vi "Digital Port Test.vi"() -> ()   [LabVIEW 2025]
doc: "Author: Scott Hannahs <sth@magnet.fsu.edu>\n\nThis software is licensed for use under the “MIT License\"\nCopyright (c) 2025 Scott Hannahs, sth@sth@magnet.sthnet.net\n\nPermission is hereby granted, free of charge, to any person obtaining a copy of this software and associated documentation files (the \"Software\"), to deal in the Software without restriction, including without limitation the rights to use, copy, modify, merge, publish, distribute, sublicense, and/or sell copies of the Software, and to permit persons to whom the Software is furnished to do so, subject to the following conditions: The above copyright notice and this permission notice shall be included in all copies or substantial portions of the Software.\n\nTHE SOFTWARE IS PROVIDED \"AS IS\", WITHOUT WARRANTY OF ANY KIND, EXPRESS OR IMPLIED, INCLUDING BUT NOT LIMITED TO THE WARRANTIES OF MERCHANTABILITY, FITNESS FOR A PARTICULAR PURPOSE AND NONINFRINGEMENT. IN NO EVENT SHALL THE AUTHORS OR COPYRIGHT HOLDERS BE LIABLE FOR ANY CLAIM, DAMAGES OR OTHER LIABILITY, WHETHER IN AN ACTION OF CONTRACT, TORT OR OTHERWISE, ARISING FROM, OUT OF OR IN CONNECTION WITH THE SOFTWARE OR THE USE OR OTHER DEALINGS IN THE SOFTWARE."
uses:
  <vilib>/Utility/error.llb/DialogType.ctl
  <vilib>/_DAQmxBase/Internals/DAQmxBase Create Channel (DO-Digital Output).vi
  <vilib>/_DAQmxBase/Internals/DAQmxBase Write (Digital U8 1Chan 1Samp).vi
panel:
  in  "stop":bool
  out "Data Read":u8 caption="Data Write" format="%02x"
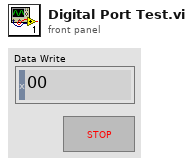
[diagram p1: front panel]
types:
  T1 = typedef "DialogType.ctl" = u16
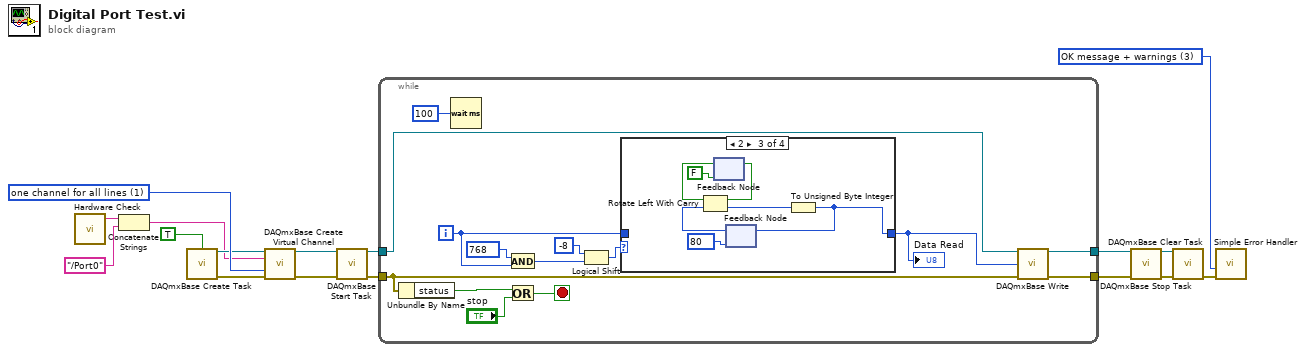
[diagram p0: block diagram]
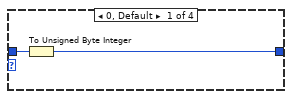
[diagram p2: hidden frame]
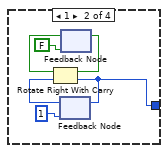
[diagram p3: hidden frame]
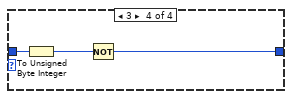
[diagram p4: hidden frame]
diagram:
  w11 = 1 items=["one channel for each line", "one channel for all lines"] ("line grouping")
  w12 = T1 3 items=["no dialog", "OK message", "continue or stop message", "OK message + warnings", "continue/stop + warnings"] ("type of dialog (OK msg:1)")
  n1 = call "Hardware Check.vi"() -> ("Data Acq Device"=w4:string)  [unwired: 1 in, 2 out]
  n2 = Concatenate Strings(w4, "/Port0" ("string")) -> (w2:string)
  n3 = call <vilib>:"DAQmxBase Create Task.vi"("auto cleanup"=TRUE) -> ("task out"=w9:refnum<k21>, "error out"=w10:errorcluster)  [unwired: 13 in]
  n4 = call-poly <vilib>:"DAQmxBase Create Virtual Channel.vi"("task in"=w9, "lines"=w2, "line grouping"=w11, "error in"=w10) -> ("task out"=w14:refnum<k21>, "error out"=w13:errorcluster)  [unwired: 10 in]
  n5 = call <vilib>:"DAQmxBase Start Task.vi"("task/channels in"=w14, "error in"=w13) -> ("task out"=w15:refnum<k21>, "error out"=w17:errorcluster)  [unwired: 12 in]
  n6 = while {
    tunnel: w17 -> [w25]
    tunnel: [w24] -> w8
    tunnel: w15 -> [w28]
    tunnel: [w26] -> w7
    i -> [w20]
    stop <- w31 stop-if-true
    n7 = Unbundle By Name(w25) -> ("status"=w29:bool)
    n8 = Wait (ms)(milliseconds to wait=u32 100) -> ()  [unwired: 1 out]
    n9 = And(x=u32 768, y=w20) -> (x .and. y?=w22:u32)
    n10 = Or(x=w29, y="stop") -> (x .or. y?=w31:bool)
    n11 = Logical Shift(y=i16 -8, x=w22) -> (x << y=w18:u32)
    n12 = case shown="2" w18 {
      tunnel: [w33 w34 w40 w47] -> w19
      tunnel: w20 -> [w32 _ _ w49]
      frame 0, Default {
        n13 = To Unsigned Byte Integer(number=w32) -> (unsigned 8bit integer=w33:u8)
      }
      frame 1 {
        n14 = feedback #1(u8 1) -> (w38:u8)
        n15 = feedback #2(FALSE ("lsb carry out")) -> (w35:bool)
        n16 = Rotate Right With Carry(2:w38, 3:w35) -> (0:w34:u8, 1:w36:bool)
        n17 = feedback-in #1(w34) -> ()
        n18 = feedback-in #2(w36) -> ()
      }
      frame 2 {
        n19 = feedback #3(FALSE ("lsb carry out")) -> (w43:bool)
        n20 = feedback #4(u8 80) -> (w45:u8)
        n21 = Rotate Left With Carry(2:w45, 3:w43) -> (0:w41:u8, 1:w42:bool)
        n22 = feedback-in #3(w42) -> ()
        n23 = To Unsigned Byte Integer(number=w41) -> (unsigned 8bit integer=w40:u8)
        n24 = feedback-in #4(w40) -> ()
      }
      frame 3 {
        n25 = To Unsigned Byte Integer(number=w49) -> (unsigned 8bit integer=w48:u8)
        n26 = Not(x=w48) -> (.not. x?=w47:u8)
      }
    }
    "Data Read" <- w19
    n27 = call-poly <vilib>:"DAQmxBase Write.vi"("task/channels in"=w28, "data"=w19, "error in"=w25) -> ("task out"=w26:refnum<k21>, "error out"=w24:errorcluster)  [unwired: 11 in]
  }
  n28 = call <vilib>:"DAQmxBase Stop Task.vi"("task/channels in"=w7, "error in"=w8) -> ("task out"=w6:refnum<k21>, "error out"=w5:errorcluster)  [unwired: 12 in]
  n29 = call <vilib>:"DAQmxBase Clear Task.vi"("task in"=w6, "error in"=w5) -> ("error out"=w16:errorcluster)  [unwired: 13 in]
  n30 = call <vilib>:"Simple Error Handler.vi"("type of dialog (OK msg:1)"=w12, "error in (no error)"=w16) -> ()  [unwired: 3 in, 5 out]
